vi "Set System Property.vi"   [LabVIEW 2020, in "SLSC.lvlib"]
uses:
  <vilib>/SLSC/SLSC.lvlib
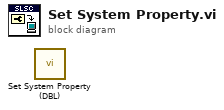
[diagram p0: block diagram]
diagram:
  n1 = call <vilib>:"Set System Property (DBL).vi"() -> ()  [unwired: 14 in, 2 out]
